vi "Macro Cluster to Text.vi"(8 "Error In":errorcluster, 11 "Macro Cluster Array IN":T1[](array[typedef])) -> (0 "Error Out":errorcluster, 2 "Argument List (Txt)":string[](array[string]), 3 "Action List (Txt)":string[](array[string]))   [LabVIEW 2012]
uses:
  Custom Controls and Typedefs/Macro_CommandStruct.ctl
  Custom Controls and Typedefs/Macro_Action_List.ctl
  Custom Controls and Typedefs/Macro_ArgumentStruct.ctl
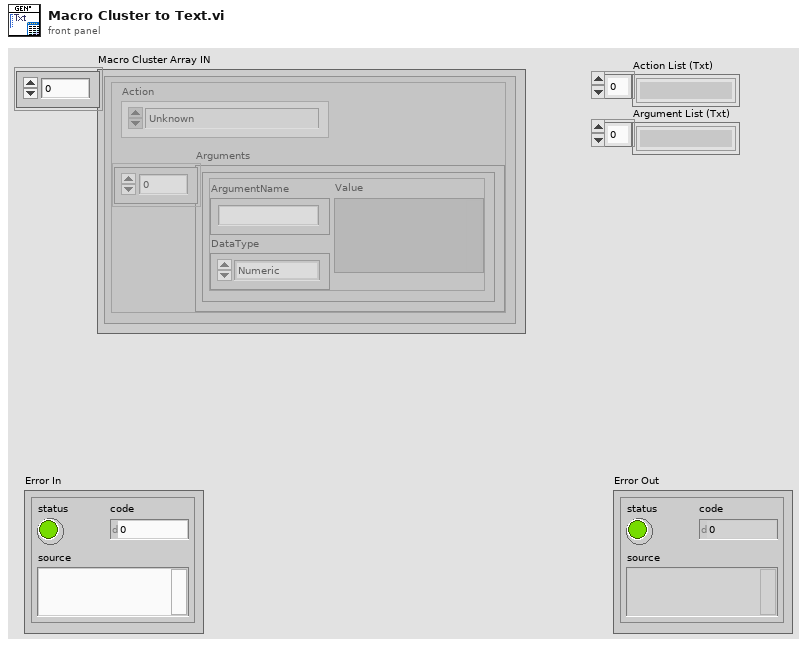
[diagram p1: front panel]
types:
  T1 = typedef "Macro_CommandStruct.ctl" = cluster{"Action":T2, "Arguments":T3[]}
  T2 = typedef "Macro_Action_List.ctl" = enum16{"Unknown", "2D.Frame.Scan", "2D.Line.Scan", "Load.Settings.File", "Move.To.Position", "Pause", "Z.Stack", "LOOP.Start", "LOOP.End"}
  T3 = typedef "Macro_ArgumentStruct.ctl" = cluster{"ArgumentName":string, "DataType":enum16{"Numeric", "String"}, "Value":variant}
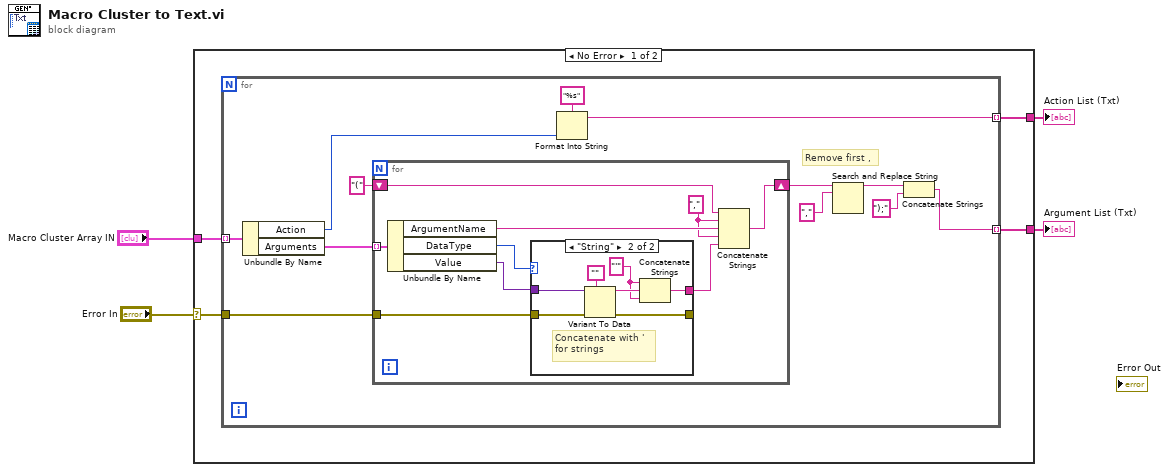
[diagram p0: block diagram]
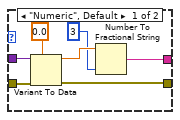
[diagram p2: hidden frame]
diagram:
  n1 = case shown="No Error" "Error In" {
    selector: "Error In" -> [w7 _]
    tunnel: "Macro Cluster Array IN" -> [w8 _]
    tunnel: [w6 _] -> w2
    tunnel: [w5 _] -> w1
    frame No Error {
      n2 = for {
        tunnel: w8 -> [w20] mode=indexing
        tunnel: w7 -> [w18]
        tunnel: [w11] -> w6 mode=indexing
        tunnel: [w10] -> w5 mode=indexing
        # "Remove first ,"
        n3 = Unbundle By Name(w20) -> ("Action"=w9:T2, "Arguments"=w19:T3[])
        n4 = for {
          tunnel: w19 -> [w29] mode=indexing
          tunnel: w18 -> [w26]
          shift-right: [w23] -> w16
          shift-left: "(" ("string") -> [w22]
          w24 = "," ("string")
          n5 = Unbundle By Name(w29) -> ("ArgumentName"=w27:string, "DataType"=w28:enum16{"Numeric", "String"}, "Value"=w21:variant)
          n6 = case shown="\"String\"" w28 {
            tunnel: w21 -> [w35 w42]
            tunnel: w26 -> [w36 w43]
            tunnel: [w30 w39] -> w25
            tunnel: [w31 w40] -> _
            frame "Numeric", Default {
              n7 = Variant To Data(error in=w36, type=0.0, Variant=w35) -> (data=w33:dbl, error out=w31:errorcluster)
              n8 = Number To Fractional String(number=w33, precision (6)=i16 3) -> (F-format string=w30:string)  [unwired: 2 in]
            }
            frame "String" {
              w37 = "'" ("string")
              # "Concatenate with '\nfor strings"
              n9 = Variant To Data(error in=w43, type="", Variant=w42) -> (data=w38:string, error out=w40:errorcluster)
              n10 = Concatenate Strings(w37, w38, w37) -> (w39:string)
            }
          }
          n11 = Concatenate Strings(w22, w24, w27, w24, w25) -> (w23:string)
        }
        n12 = Format Into String(format string="%s", w9) -> (resulting string=w11:string)  [unwired: 2 in, 1 out]
        n13 = Search and Replace String(input string=w16, search string=",") -> (result string=w14:string)  [unwired: 6 in, 3 out]
        n14 = Concatenate Strings(w14, ");" ("string")) -> (w10:string)
      }
    }
    frame Error {
    }
  }
  "Action List (Txt)" <- w2
  "Argument List (Txt)" <- w1
